vi "FunctionGenerator.vi"() -> ()   [LabVIEW 2012]
doc: "This VI illustrates how to generate and play sine, square, sawtooth and triangle waveforms. You can change the frequency and type of the waveform generated as it plays continuously."
uses:
  <vilib>/sound2/lvsound2.llb/Sound Data Format.ctl
  <vilib>/sound2/lvsound2.llb/Sampling Mode.ctl
  <vilib>/sound2/lvsound2.llb/Sound Output Set Volume (Single).vi
  <vilib>/sound2/lvsound2.llb/Sound Output Write (DBL Single).vi
  <vilib>/measure/NI_MABase.lvlib
panel:
  in  "Volume":dbl=70.0 step=0.01
  in  "Sound Format":T1={"sample rate (S/s)"=44100.0, "number of channels"=2, "bits per sample"=16}
  out "Generated Sound":waveform(dbl)(graph)={"t0"=timestamp(1.2471655328798186 s since 1904-01-01), "dt"=2.2675736961451248e-05, "Y"=[]}
  in  "Waveform Type":enum16{"Sine", "Square", "Sawtooth", "Triangle"}(ring)
  in  "Frequency":dbl=2500.0 format="%0.2p"
  in  "stop":bool
  in  "Number of Samples/ch":i32=5000
  in  "Device ID":u32
  # "Configuration"
  # "This VI illustrates how to generate and play sine, square, sawtooth and triangle waveforms continuously. \n\nInstructions to execute the VI:\n1.  Specify Device ID, bits per sample, sample rate and number of samples (buffer size).\n2.  Select the waveform type to play and its initial frequency.\n3.  Run the VI. Waveforms are generated and sent to both the graph and your speakers.\n3.  Change the frequency to change the pitch of the sound.\n4.  Change the waveform type to start playing differently shaped waves.\n5.  Press the stop button when done.\n100% setting                                                 80% setting\nVmax peak to peak = 3.62-3.66V                Vmax peak to peak = 1.82V - 1.84V\nVmax = 1.84V                                                Vmax = 0.92V\nVmin = -1.82                                                 Vmin = -0.90V\n\n70% setting                                                   50% setting\nVmax peak to peak = 1.06V - 1.09V           Vmax peak to peak ~ 300mV\nVmax = 0.536V                                             Vmax ~ 140mV\nVmin = -0.552V                                            Vmin ~ -156mV"
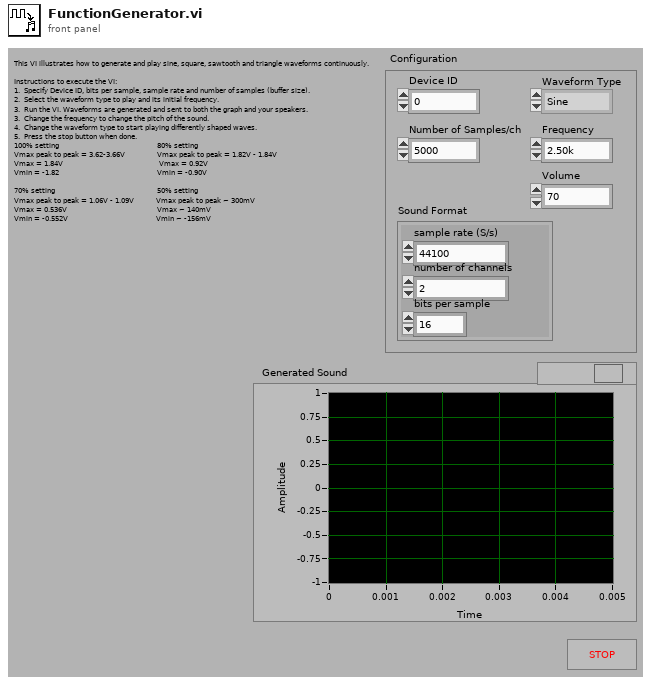
[diagram p1: front panel]
types:
  T1 = typedef "Sound Data Format.ctl" = cluster{"sample rate (S/s)":dbl, "number of channels":i32, "bits per sample":i32}
  T2 = typedef "Sampling Mode.ctl" = i32
  T3 = typedef "Sound Output Task ID.ctl" = u32
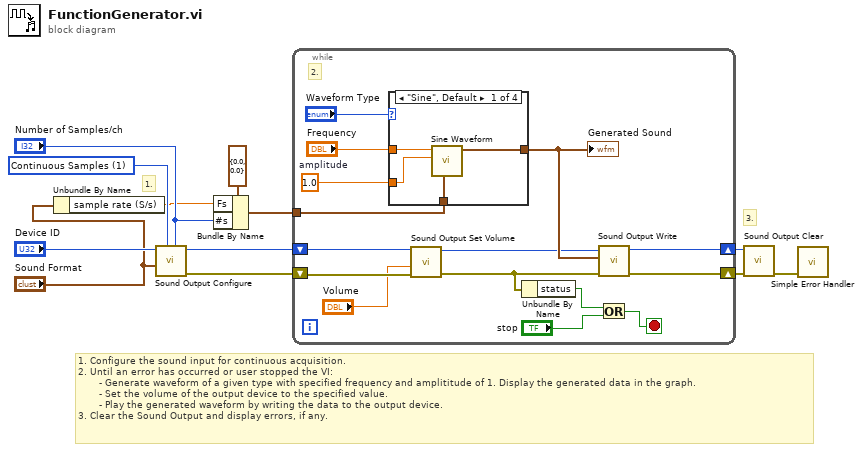
[diagram p0: block diagram]
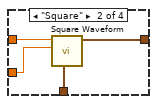
[diagram p2: hidden frame]
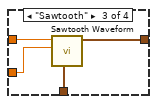
[diagram p3: hidden frame]
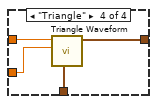
[diagram p4: hidden frame]
diagram:
  w7 = T2 1 items=["Finite Samples", "Continuous Samples"] ("sample mode")
  # "3."
  # "1."
  # "1. Configure the sound input for continuous acquisition.\n2. Until an error has occurred or user stopped the VI: \n      \t- Generate waveform of a given type with specified frequency and amplititude of 1. Display the generated data in the graph. \n       - Set the volume of the output device to the specified value.\n      \t- Play the generated waveform by writing the data to the output device.\n3. Clear the Sound Output and display errors, if any."
  n1 = Unbundle By Name("Sound Format") -> ("sample rate (S/s)"=w2:dbl)
  n2 = call <vilib>:"Sound Output Configure.vi"("number of samples/ch"="Number of Samples/ch", "sample mode"=w7, "sound format"="Sound Format", "device ID"="Device ID") -> ("error out"=w12:errorcluster, "task ID"=w11:T3)  [unwired: 6 in]
  n3 = Bundle By Name(cluster=cluster{"Fs":dbl, "#s":dbl} {"Fs"=0.0, "#s"=0.0} ("sampling info"), "Fs"=w2, "#s"="Number of Samples/ch") -> (w4:cluster{"Fs":dbl, "#s":dbl})
  n4 = while {
    shift-right: [w26] -> w10
    shift-left: w12 -> [w16]
    shift-right: [w27] -> w9
    shift-left: w11 -> [w14]
    tunnel: w4 -> [w21]
    stop <- w24 stop-if-true
    w19 = 1.0  # amplitude
    # "2."
    n5 = case shown="\"Sine\", Default" "Waveform Type" {
      tunnel: "Frequency" -> [w31 w34 w36 w43]
      tunnel: [w30 w33 w38 w42] -> w18
      tunnel: w21 -> [w29 w35 w39 w41]
      tunnel: w19 -> [w28 w32 w37 w40]
      frame "Sine", Default {
        n6 = call <vilib>:"Sine Waveform.vi"("sampling info"=w29, "amplitude"=w28, "frequency"=w31) -> ("signal out"=w30:waveform(dbl))  [unwired: 7 in, 1 out]
      }
      frame "Square" {
        n7 = call <vilib>:"Square Waveform.vi"("sampling info"=w35, "amplitude"=w32, "frequency"=w34) -> ("signal out"=w33:waveform(dbl))  [unwired: 7 in, 1 out]
      }
      frame "Sawtooth" {
        n8 = call <vilib>:"Sawtooth Waveform.vi"("sampling info"=w39, "amplitude"=w37, "frequency"=w36) -> ("signal out"=w38:waveform(dbl))  [unwired: 7 in, 1 out]
      }
      frame "Triangle" {
        n9 = call <vilib>:"Triangle Waveform.vi"("sampling info"=w41, "amplitude"=w40, "frequency"=w43) -> ("signal out"=w42:waveform(dbl))  [unwired: 7 in, 1 out]
      }
    }
    "Generated Sound" <- w18
    n10 = call-poly <vilib>:"Sound Output Set Volume.vi"("error in (no error)"=w16, "volume"="Volume", "task ID"=w14) -> ("error out"=w17:errorcluster, "task ID out"=w15:T3)  [unwired: 7 in]
    n11 = Unbundle By Name(w17) -> ("status"=w22:bool)
    n12 = call-poly <vilib>:"Sound Output Write.vi"("error in (no error)"=w17, "data"=w18, "task ID"=w15) -> ("error out"=w26:errorcluster, "task ID out"=w27:T3)  [unwired: 7 in]
    n13 = Or(x=w22, y="stop") -> (x .or. y?=w24:bool)
  }
  n14 = call <vilib>:"Sound Output Clear.vi"("error in (no error)"=w10, "task ID"=w9) -> ("error out"=w3:errorcluster)  [unwired: 9 in]
  n15 = call <vilib>:"Simple Error Handler.vi"("error in (no error)"=w3) -> ()  [unwired: 4 in, 5 out]
